vi "Update.vi"(6 "Assembly Type":string, 7 "Row":i32, 8 "error in (no error)":errorcluster, 9 "Workspace":T1, 10 "Routine":T2=enum."Dispense Epoxy", 11 "Assembly Run in":refnum<class "Assembly Run.lvclass">) -> (0 "error out":errorcluster, 3 "Assembly Run out":refnum<class "Assembly Run.lvclass">)   [LabVIEW 2021, in "Assembly Run.lvclass"]
uses:
  Assembly Run.lvclass
  Routine/Routine Enum.ctl
  Workspace/Fixture Enum.ctl
  Assembly Run.lvclass/Assembly Run.ctl
  Routine/Routine.lvclass
  Workspace/Fixture.lvclass
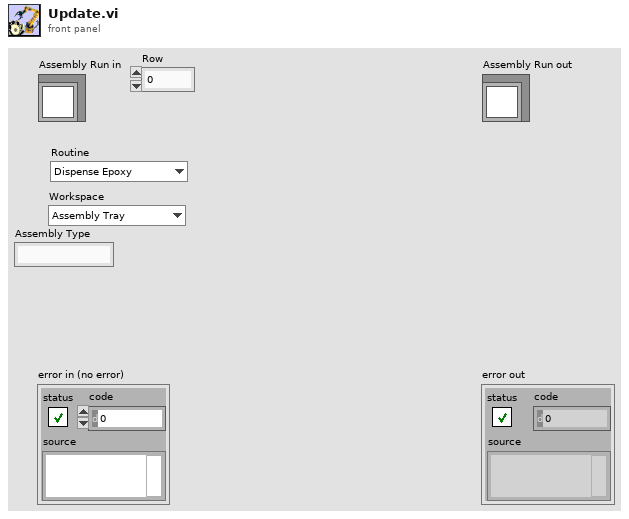
[diagram p1: front panel]
types:
  T1 = typedef "Fixture.lvclass/Fixture Enum.ctl" = enum16{"Assembly Tray", "Syringe Space", "Component", "Pick Up Tool", "Current Position"}
  T2 = typedef "Routine.lvclass/Routine Enum.ctl" = enum16{"Primary Pick Up", "Secondary Pick Up", "Put Down All", "Secure Syringe", "Release Syringe", "Dispense Epoxy", "Pick Up All", "Put Down Secondary", "Full Assembly"}
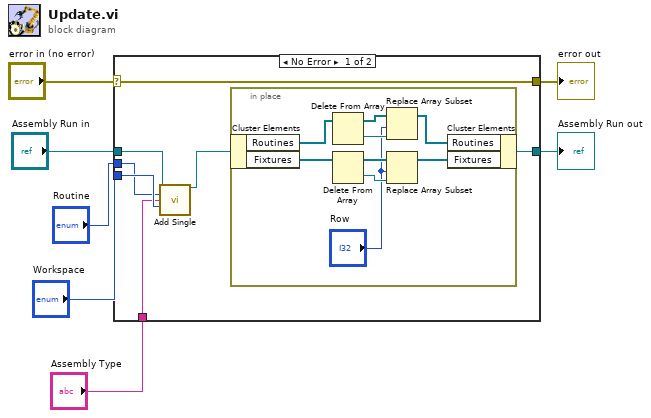
[diagram p0: block diagram]
diagram:
  n1 = case shown="No Error" "error in (no error)" {
    selector: "error in (no error)" -> [w14 w25]
    tunnel: [w14 w25] -> w6
    tunnel: [w13 w24] -> w4
    tunnel: "Assembly Run in" -> [w11 w24]
    tunnel: "Routine" -> [w9 _]
    tunnel: "Workspace" -> [w12 _]
    tunnel: "Assembly Type" -> [w8 _]
    frame No Error {
      n2 = call-dynamic "Add Single.vi"("UI in"=w11, "Routine"=w9, "Assembly Type"=w8, "Fixture"=w12) -> ("UI out"=w10:refnum<class "Assembly Run.lvclass">)  [unwired: 10 in, 1 out]
      n3 = in-place {
        n4 = in-place-cluster #1(w10) -> ("Routines"=w19:refnum<class "Routine.lvclass">[], "Fixtures"=w18:refnum<class "Fixture.lvclass">[])
        n5 = Delete From Array(array=w19) -> (deleted portion=w21:refnum<class "Routine.lvclass">, array with subset deleted=w20:refnum<class "Routine.lvclass">[])  [unwired: 2 in]
        n6 = Delete From Array(array=w18) -> (deleted portion=w22:refnum<class "Fixture.lvclass">, array with subset deleted=w23:refnum<class "Fixture.lvclass">[])  [unwired: 2 in]
        n7 = Replace Array Subset(array=w20, new element=w21, index="Row") -> (w17:refnum<class "Routine.lvclass">[])
        n8 = Replace Array Subset(array=w23, new element=w22, index="Row") -> (w16:refnum<class "Fixture.lvclass">[])
        n9 = in-place-cluster #1("Routines"=w17, "Fixtures"=w16) -> (w13:refnum<class "Assembly Run.lvclass">)
      }
    }
    frame Error {
    }
  }
  "error out" <- w6
  "Assembly Run out" <- w4
